vi "Set Value.vi"(8 "error in (no error)":errorcluster, 10 "value":string, 11 "SingleB in":refnum<class "SingleB.lvclass">) -> (0 "error out":errorcluster, 3 "SingleB out":refnum<class "SingleB.lvclass">)   [LabVIEW 2020, in "SingleB.lvclass"]
uses:
  SingleB.lvclass
  D:/03 GitHub/LabVIEW-Singleton/Singleton/Singleton.lvclass
  Singleton/Singleton.lvclass/Singleton.ctl
  SingleB.lvclass/SingleB.ctl
  Singleton/Singleton.lvclass
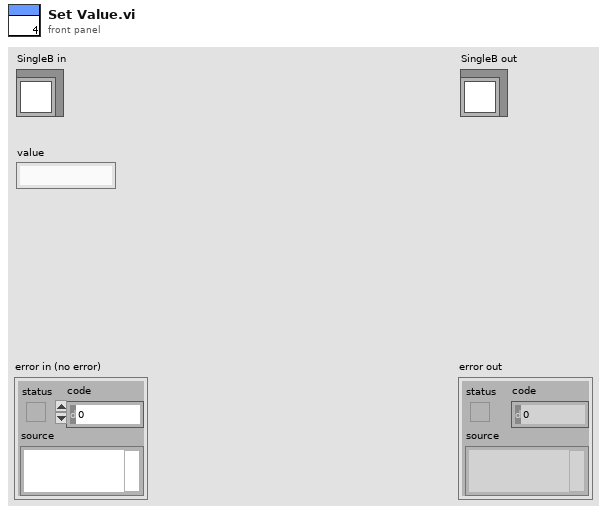
[diagram p1: front panel]
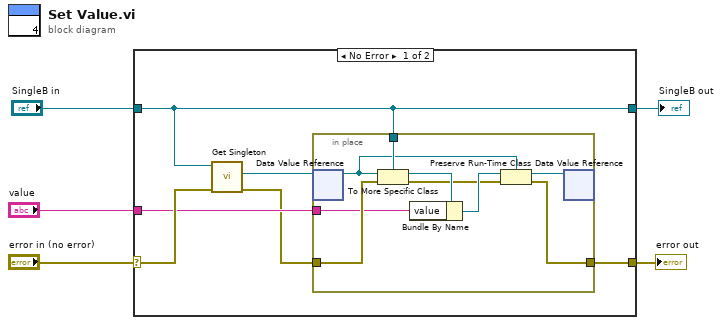
[diagram p0: block diagram]
diagram:
  n1 = case shown="No Error" "error in (no error)" {
    selector: "error in (no error)" -> [w9 w22]
    tunnel: [w8 w22] -> w4
    tunnel: [w10 w21] -> w2
    tunnel: "SingleB in" -> [w10 w21]
    tunnel: "value" -> [w7 _]
    frame No Error {
      n2 = call "Get Singleton.vi"("error in (no error)"=w9, "Singleton in"=w10) -> ("error out"=w6:errorcluster, "singleton"=w11:refnum<data-value>)  [unwired: 7 in, 1 out]
      n3 = in-place {
        in-place-border: w10 -> [w20]
        in-place-border: w6 -> [w15]
        in-place-border: [w13] -> w8
        in-place-border: w7 -> [w12]
        n4 = in-place-dvr #1(w11) -> (w19:refnum<class>)  [unwired: 1 out]
        n5 = To More Specific Class(target class=w20, reference=w19, error in=w15) -> (specific class reference=w17:refnum<class "SingleB.lvclass">, error out=w14:errorcluster)
        n6 = Bundle By Name(cluster=w17, "value"=w12) -> (w16:refnum<class "SingleB.lvclass">)
        n7 = Preserve Run-Time Class(object in=w16, error in=w14, 2:w19) -> (object out=w18:refnum<class>, error out=w13:errorcluster)
        n8 = in-place-dvr #1(w18) -> ()  [unwired: 2 out]
      }
    }
    frame Error {
    }
  }
  "error out" <- w4
  "SingleB out" <- w2
